vi "SSC Digital Configure Single Level.vi"(0 "Digital SSC in":T1[](array[typedef]), 5 "Level Type to Set":T2, 7 "Setting":dbl, 11 "error in":errorcluster) -> (4 "Digital SSC out":T1[](array[typedef]), 15 "error out":errorcluster)   [LabVIEW 2020]
doc: "Configures and applies the specified single level to the specified pin(s) and pin group(s)."
uses:
  SSC Digital Single Level Selection.ctl
  SSC Digital.ctl
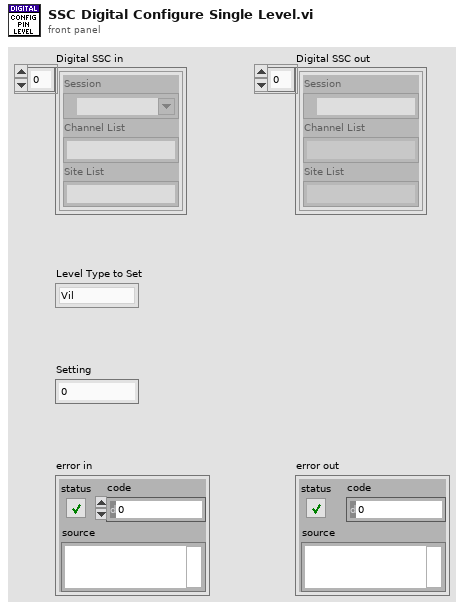
[diagram p1: front panel]
types:
  T1 = typedef "SSC Digital.ctl" = cluster{"Session":refnum<k15>, "Channel List":string, "Site List":string}
  T2 = typedef "SSC Digital Single Level Selection.ctl" = enum16{"Vil", "Vih", "Vol", "Voh", "Vterm", "Iol", "Ioh", "Vcom"}
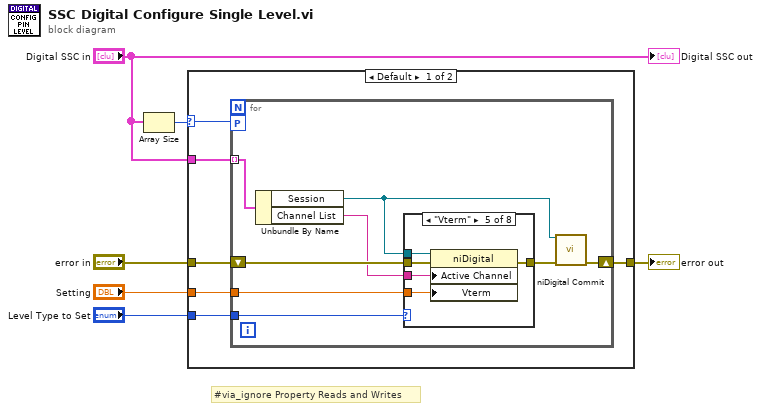
[diagram p0: block diagram]
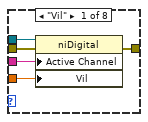
[diagram p2: hidden frame]
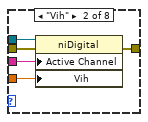
[diagram p3: hidden frame]
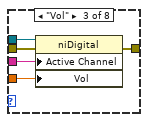
[diagram p4: hidden frame]
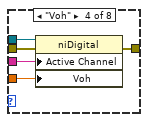
[diagram p5: hidden frame]
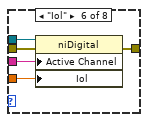
[diagram p6: hidden frame]
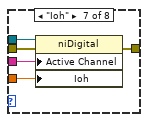
[diagram p7: hidden frame]
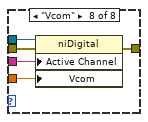
[diagram p8: hidden frame]
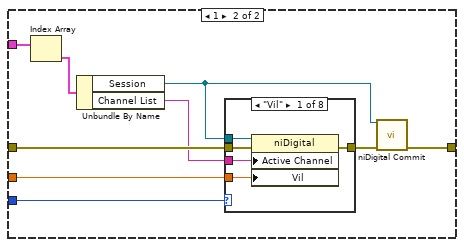
[diagram p9: hidden frame]
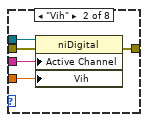
[diagram p10: hidden frame]
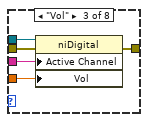
[diagram p11: hidden frame]
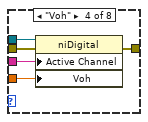
[diagram p12: hidden frame]
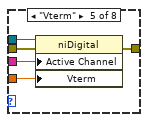
[diagram p13: hidden frame]
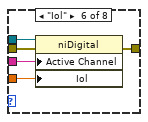
[diagram p14: hidden frame]
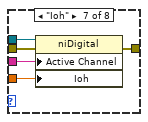
[diagram p15: hidden frame]
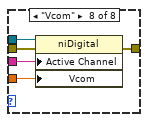
[diagram p16: hidden frame]
diagram:
  # "#via_ignore Property Reads and Writes"
  n1 = Array Size(array="Digital SSC in") -> (size(s)=w2:i32)
  n2 = case shown="Default" w2 {
    selector: w2 -> [w8 _]
    tunnel: "Setting" -> [w12 w69]
    tunnel: "Level Type to Set" -> [w11 w68]
    tunnel: "error in" -> [w10 w67]
    tunnel: [w9 w66] -> w3
    tunnel: "Digital SSC in" -> [w7 w65]
    frame Default {
      n3 = for {
        workers-P: w8 -> [_]
        tunnel: w12 -> [w17]
        tunnel: w11 -> [w16]
        tunnel: w7 -> [w15] mode=indexing
        shift-right: [w18] -> w9
        shift-left: w10 -> [w20]
        n4 = Unbundle By Name(w15) -> ("Session"=w14:refnum<k15>, "Channel List"=w13:string)
        n5 = case shown="\"Vterm\"" w16 {
          tunnel: w20 -> [w25 w30 w35 w40 w45 w50 w55 w60]
          tunnel: [w24 w29 w34 w39 w44 w49 w54 w59] -> w19
          tunnel: w14 -> [w23 w28 w33 w38 w43 w48 w53 w58]
          tunnel: w13 -> [w22 w27 w32 w37 w42 w47 w52 w57]
          tunnel: w17 -> [w21 w26 w31 w36 w41 w46 w51 w56]
          frame "Vil" {
            n6 = property on="Property Node" class="niDigital"(reference=w23, error in=w25, "Active Channel"=w22, "Vil"=w21) -> (error out=w24:errorcluster)  [unwired: 1 out]
          }
          frame "Vih" {
            n7 = property on="Property Node" class="niDigital"(reference=w28, error in=w30, "Active Channel"=w27, "Vih"=w26) -> (error out=w29:errorcluster)  [unwired: 1 out]
          }
          frame "Vol" {
            n8 = property on="Property Node" class="niDigital"(reference=w33, error in=w35, "Active Channel"=w32, "Vol"=w31) -> (error out=w34:errorcluster)  [unwired: 1 out]
          }
          frame "Voh" {
            n9 = property on="Property Node" class="niDigital"(reference=w38, error in=w40, "Active Channel"=w37, "Voh"=w36) -> (error out=w39:errorcluster)  [unwired: 1 out]
          }
          frame "Vterm" {
            n10 = property on="Property Node" class="niDigital"(reference=w43, error in=w45, "Active Channel"=w42, "Vterm"=w41) -> (error out=w44:errorcluster)  [unwired: 1 out]
          }
          frame "Iol" {
            n11 = property on="Property Node" class="niDigital"(reference=w48, error in=w50, "Active Channel"=w47, "Iol"=w46) -> (error out=w49:errorcluster)  [unwired: 1 out]
          }
          frame "Ioh" {
            n12 = property on="Property Node" class="niDigital"(reference=w53, error in=w55, "Active Channel"=w52, "Ioh"=w51) -> (error out=w54:errorcluster)  [unwired: 1 out]
          }
          frame "Vcom" {
            n13 = property on="Property Node" class="niDigital"(reference=w58, error in=w60, "Active Channel"=w57, "Vcom"=w56) -> (error out=w59:errorcluster)  [unwired: 1 out]
          }
        }
        n14 = call <instrlib>:"niDigital Commit.vi"("instrument handle"=w14, "error in"=w19) -> ("error out"=w18:errorcluster)  [unwired: 12 in, 1 out]
      }
    }
    frame 1 {
      n15 = Index Array(array=w65) -> (element=w61:T1)  [unwired: 1 in]
      n16 = Unbundle By Name(w61) -> ("Session"=w63:refnum<k15>, "Channel List"=w62:string)
      n17 = case shown="\"Vil\"" w68 {
        tunnel: w67 -> [w74 w79 w84 w89 w94 w99 w104 w109]
        tunnel: [w73 w78 w83 w88 w93 w98 w103 w108] -> w64
        tunnel: w63 -> [w72 w77 w82 w87 w92 w97 w102 w107]
        tunnel: w62 -> [w71 w76 w81 w86 w91 w96 w101 w106]
        tunnel: w69 -> [w70 w75 w80 w85 w90 w95 w100 w105]
        frame "Vil" {
          n18 = property on="Property Node" class="niDigital"(reference=w72, error in=w74, "Active Channel"=w71, "Vil"=w70) -> (error out=w73:errorcluster)  [unwired: 1 out]
        }
        frame "Vih" {
          n19 = property on="Property Node" class="niDigital"(reference=w77, error in=w79, "Active Channel"=w76, "Vih"=w75) -> (error out=w78:errorcluster)  [unwired: 1 out]
        }
        frame "Vol" {
          n20 = property on="Property Node" class="niDigital"(reference=w82, error in=w84, "Active Channel"=w81, "Vol"=w80) -> (error out=w83:errorcluster)  [unwired: 1 out]
        }
        frame "Voh" {
          n21 = property on="Property Node" class="niDigital"(reference=w87, error in=w89, "Active Channel"=w86, "Voh"=w85) -> (error out=w88:errorcluster)  [unwired: 1 out]
        }
        frame "Vterm" {
          n22 = property on="Property Node" class="niDigital"(reference=w92, error in=w94, "Active Channel"=w91, "Vterm"=w90) -> (error out=w93:errorcluster)  [unwired: 1 out]
        }
        frame "Iol" {
          n23 = property on="Property Node" class="niDigital"(reference=w97, error in=w99, "Active Channel"=w96, "Iol"=w95) -> (error out=w98:errorcluster)  [unwired: 1 out]
        }
        frame "Ioh" {
          n24 = property on="Property Node" class="niDigital"(reference=w102, error in=w104, "Active Channel"=w101, "Ioh"=w100) -> (error out=w103:errorcluster)  [unwired: 1 out]
        }
        frame "Vcom" {
          n25 = property on="Property Node" class="niDigital"(reference=w107, error in=w109, "Active Channel"=w106, "Vcom"=w105) -> (error out=w108:errorcluster)  [unwired: 1 out]
        }
      }
      n26 = call <instrlib>:"niDigital Commit.vi"("instrument handle"=w63, "error in"=w64) -> ("error out"=w66:errorcluster)  [unwired: 12 in, 1 out]
    }
  }
  "error out" <- w3
  "Digital SSC out" <- "Digital SSC in"
